vi "Handle TCP Message.vi"(7 "TCPMessageAPI":refnum<class "TCPMessageAPI.lvclass">, 8 "error in (no error)":errorcluster, 10 "TcpPayload":T1, 11 "RequestReply Message Handler in":refnum<class "RequestReply Message Handler.lvclass">) -> (0 "error out":errorcluster, 3 "RequestReply Message Handler out":refnum<class "RequestReply Message Handler.lvclass">)   [LabVIEW 2020, in "VectoScratch.lvlib" / "RequestReply Message Handler.lvclass"]
uses:
  RequestReply Message Handler.lvclass
  Vecto/TCPMessageService/TCPMessageAPI.lvclass
  lv-volatus/messages/TcpPayload/Data.ctl
  RequestReply Message Handler.lvclass/RequestReply Message Handler.ctl
  proto/messages/RequestTwoDouble/RequestTwoDouble.lvlib
  proto/messages/ReplyOneDouble/ReplyOneDouble.lvlib
  lv-volatus/messages/TcpPayload/TcpPayload.lvlib
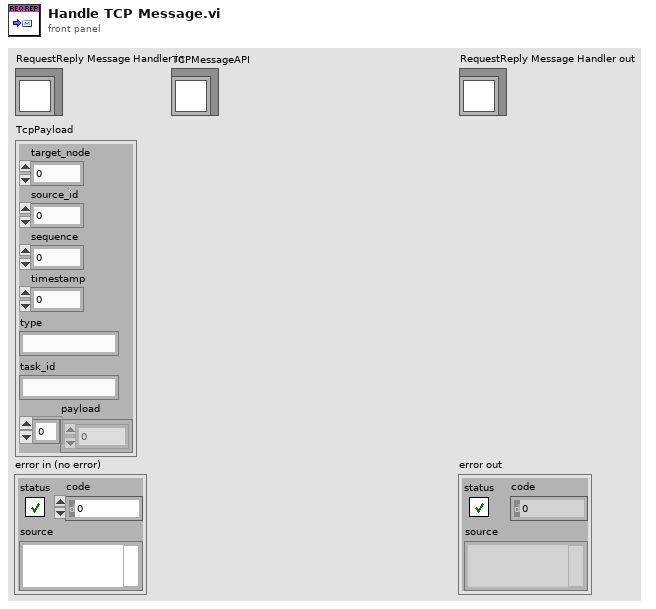
[diagram p1: front panel]
types:
  T1 = typedef "TcpPayload.lvlib/Data.ctl" = cluster{"target_node":u32, "source_id":u32, "sequence":u32, "timestamp":i64, "type":string, "task_id":string, "payload":u8[]}
  T2 = typedef "RequestTwoDouble.lvlib/Data.ctl" = cluster{"a":dbl, "b":dbl}
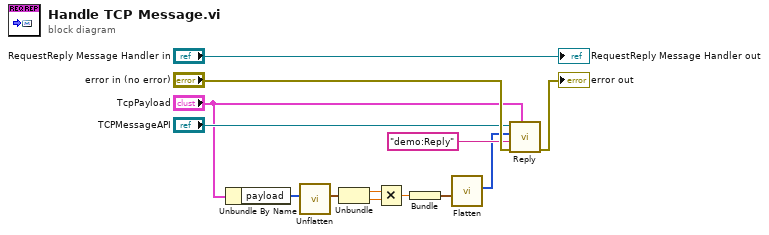
[diagram p0: block diagram]
diagram:
  n1 = Unbundle By Name("TcpPayload") -> ("payload"=w5:u8[])
  n2 = call "Unflatten.vi"("Buffer"=w5) -> ("Data"=w4:T2)  [unwired: 9 in, 1 out]
  n3 = Unbundle(w4) -> ("a"=w11:dbl, "b"=w10:dbl)
  n4 = Multiply(x=w11, y=w10) -> (x*y=w3:dbl)
  n5 = Bundle(w3) -> (w2:cluster{dbl})  [unwired: 1 in]
  n6 = call "Flatten.vi"("Data"=w2) -> ("Buffer"=w1:u8[])  [unwired: 9 in, 1 out]
  n7 = call "Reply.vi"("Original Payload"="TcpPayload", "error in (no error)"="error in (no error)", "Type"="demo:Reply", "Payload"=w1, "TCPMessageAPI in"="TCPMessageAPI") -> ("error out"=→"error out":errorcluster)  [unwired: 5 in, 1 out]
  "RequestReply Message Handler out" <- "RequestReply Message Handler in"
